vi "RPC_DAQ.vi"(7 "address":string[](array[string])=["192.168.10.20"], 8 "error in (no error)":errorcluster, 9 "stop":bool, 10 "save data":bool=TRUE, 11 "SMA mode":bool) -> (0 "error out 3":errorcluster, 2 "csv path":path=path "G:/tdc/2017/data/test_20250729_102001.csv", 3 "rate":dbl=0.9690537851551113)   [LabVIEW 2017]
uses:
  gloabal.vi
  <vilib>/Utility/file.llb/Write Delimited Spreadsheet (DBL).vi
  <vilib>/Utility/file.llb/Write Delimited Spreadsheet (I64).vi
panel:
  in  "index (row)":i32
  out "fine":u64
  out "Array 2":u64[](array[numeric])
  out "PAD":u64
  out "hitmap":u64=2 format="%08b"
  out "name (unnamed) 4":string
  out "name (unnamed) 3":string
  out "name (unnamed) 2":string
  out "Array":string[](array[string])
  out "pmt trigger rate":u32[](array[numeric])=[0, 59394, 0, 0, 0, 0, 0, 0, 0, 0, 0, 0, 0, 0, 0, 0, 0, 0, 0, 0, 0, 0, 0, 0, 0, 0, 0, 0, 0, 0, 0, 0, 0, 0, 0, 0, 0, 59424, 0, 0, 0, 0, 0, 0, 0, 0, 0, 0, 0, 0, 0, 0, 0, 0, 0, 0, 0, 0, 0, 0, 0, 0, 0, 0, 0, 0, 0, 0, 0, 0, 0, 0, 0, 0, 0, 0, 0, 0, 0, 0, 0, 0, 0, 0, 0, 0, 0, 0, 0, 0, 0, 0, 0, 0, 0, 0, 0, 0, 0, 0, 0, 0, 0, 0, 0, 0, 0, 0, 0, 0, 0, 0, 0, 0, 0, 0, 0, 0, 0, 0, 0, 0, 0, 0, 0, 0, 0, 0]
  out "event":u32[](array[numeric])=[0, 1657, 0, 0, 0, 0, 0, 0, 0, 0, 0, 0, 0, 0, 0, 0, 0, 0, 0, 0, 0, 0, 0, 0, 0, 0, 0, 0, 0, 0, 0, 0, 0, 0, 0, 0, 0, 863, 0, 0, 0, 0, 0, 0, 0, 0, 0, 0, 0, 0, 0, 0, 0, 0, 0, 0, 0, 0, 0, 0, 0, 0, 0, 0, 0, 0, 0, 0, 0, 0, 0, 0, 0, 0, 0, 0, 0, 0, 0, 0, 0, 0, 0, 0, 0, 0, 0, 0, 0, 0, 0, 0, 0, 0, 0, 0, 0, 0, 0, 0, 0, 0, 0, 0, 0, 0, 0, 0, 0, 0, 0, 0, 0, 0, 0, 0, 0, 0, 0, 0, 0, 0, 0, 0, 0, 0, 0, 0]
  in  "calib_file":path=path "G:/tdc/2017/data/112_20250410_codeDensity.csv" caption="文件路径 （空时为对话框）"
  in  "use_calib_file":bool
  in  "coarse counter width":u16(ring) items=["29", "48"]
  out "name (unnamed)":string
  out "error out 5":errorcluster
  in  "timeout":dbl=30000.0
  out "DAC":dbl=8094.0
  out "Out":u8=3 format="%.0x"
  in  "gps":bool
  out "Year":string="2025"
  in  "factor":i32=128
  in  "displayCR":bool=TRUE
  in  "Counter Setting":dbl=100000.0 format="%#_13g"
  in  "replace dat":bool
  in  "append csv":bool=TRUE
  out "element":string
  out "time":u64=1569737306459 format="%x"
  in  "UDP Config":bool
  in  "data  path":path=path "G:/tdc/2017/data"
  out "cal 2":u64[](graph)
  in  "Thresholds (mV)":dbl[](array[numeric])=[580.0, 580.0, 580.0, 580.0, 600.0, 600.0, 600.0, 600.0, 580.0, 580.0, 600.0, 600.0, 600.0, 600.0, 600.0, 600.0, 580.0, 580.0, 600.0, 600.0, 600.0, 600.0, 600.0, 600.0, 580.0, 580.0, 600.0, 600.0, 600.0, 600.0, 600.0, 600.0, 600.0, 600.0, 600.0, 600.0, 600.0, 600.0, 600.0, 600.0, 600.0, 600.0, 600.0, 600.0, 600.0, 600.0, 600.0, 600.0, 600.0, 600.0, 600.0, 600.0, 600.0, 600.0, 600.0, 600.0, 600.0, 600.0, 600.0, 600.0, 600.0, 600.0, 600.0, 600.0]
  out "error out 2":errorcluster
  in  "display":bool=TRUE
  in  "Thresholds":dbl=-0.03
  in  "one key for threshold":bool=TRUE
  in  "RST":bool
  in  "通道数量":i32=128
  out "Cal Table":u32[](array[numeric])
  in  "channel for cal":i32
  out "channel number":u64=1
  out "Calibration Counter":i32=3364
  out "Event index":i32=97959
  out "cal":i64[](graph)
  out "error out":errorcluster={"status"=TRUE, "code"=1, "source"="Close File in RPC_DAQ.vi"}
  out "appended path":path=path "G:/tdc/2017/data/test_20250729_102001.dat"
  in  "filename":string="test"
  in  "Events":i32=110000 min=1
  in  "timeout (ms)":i32=10000
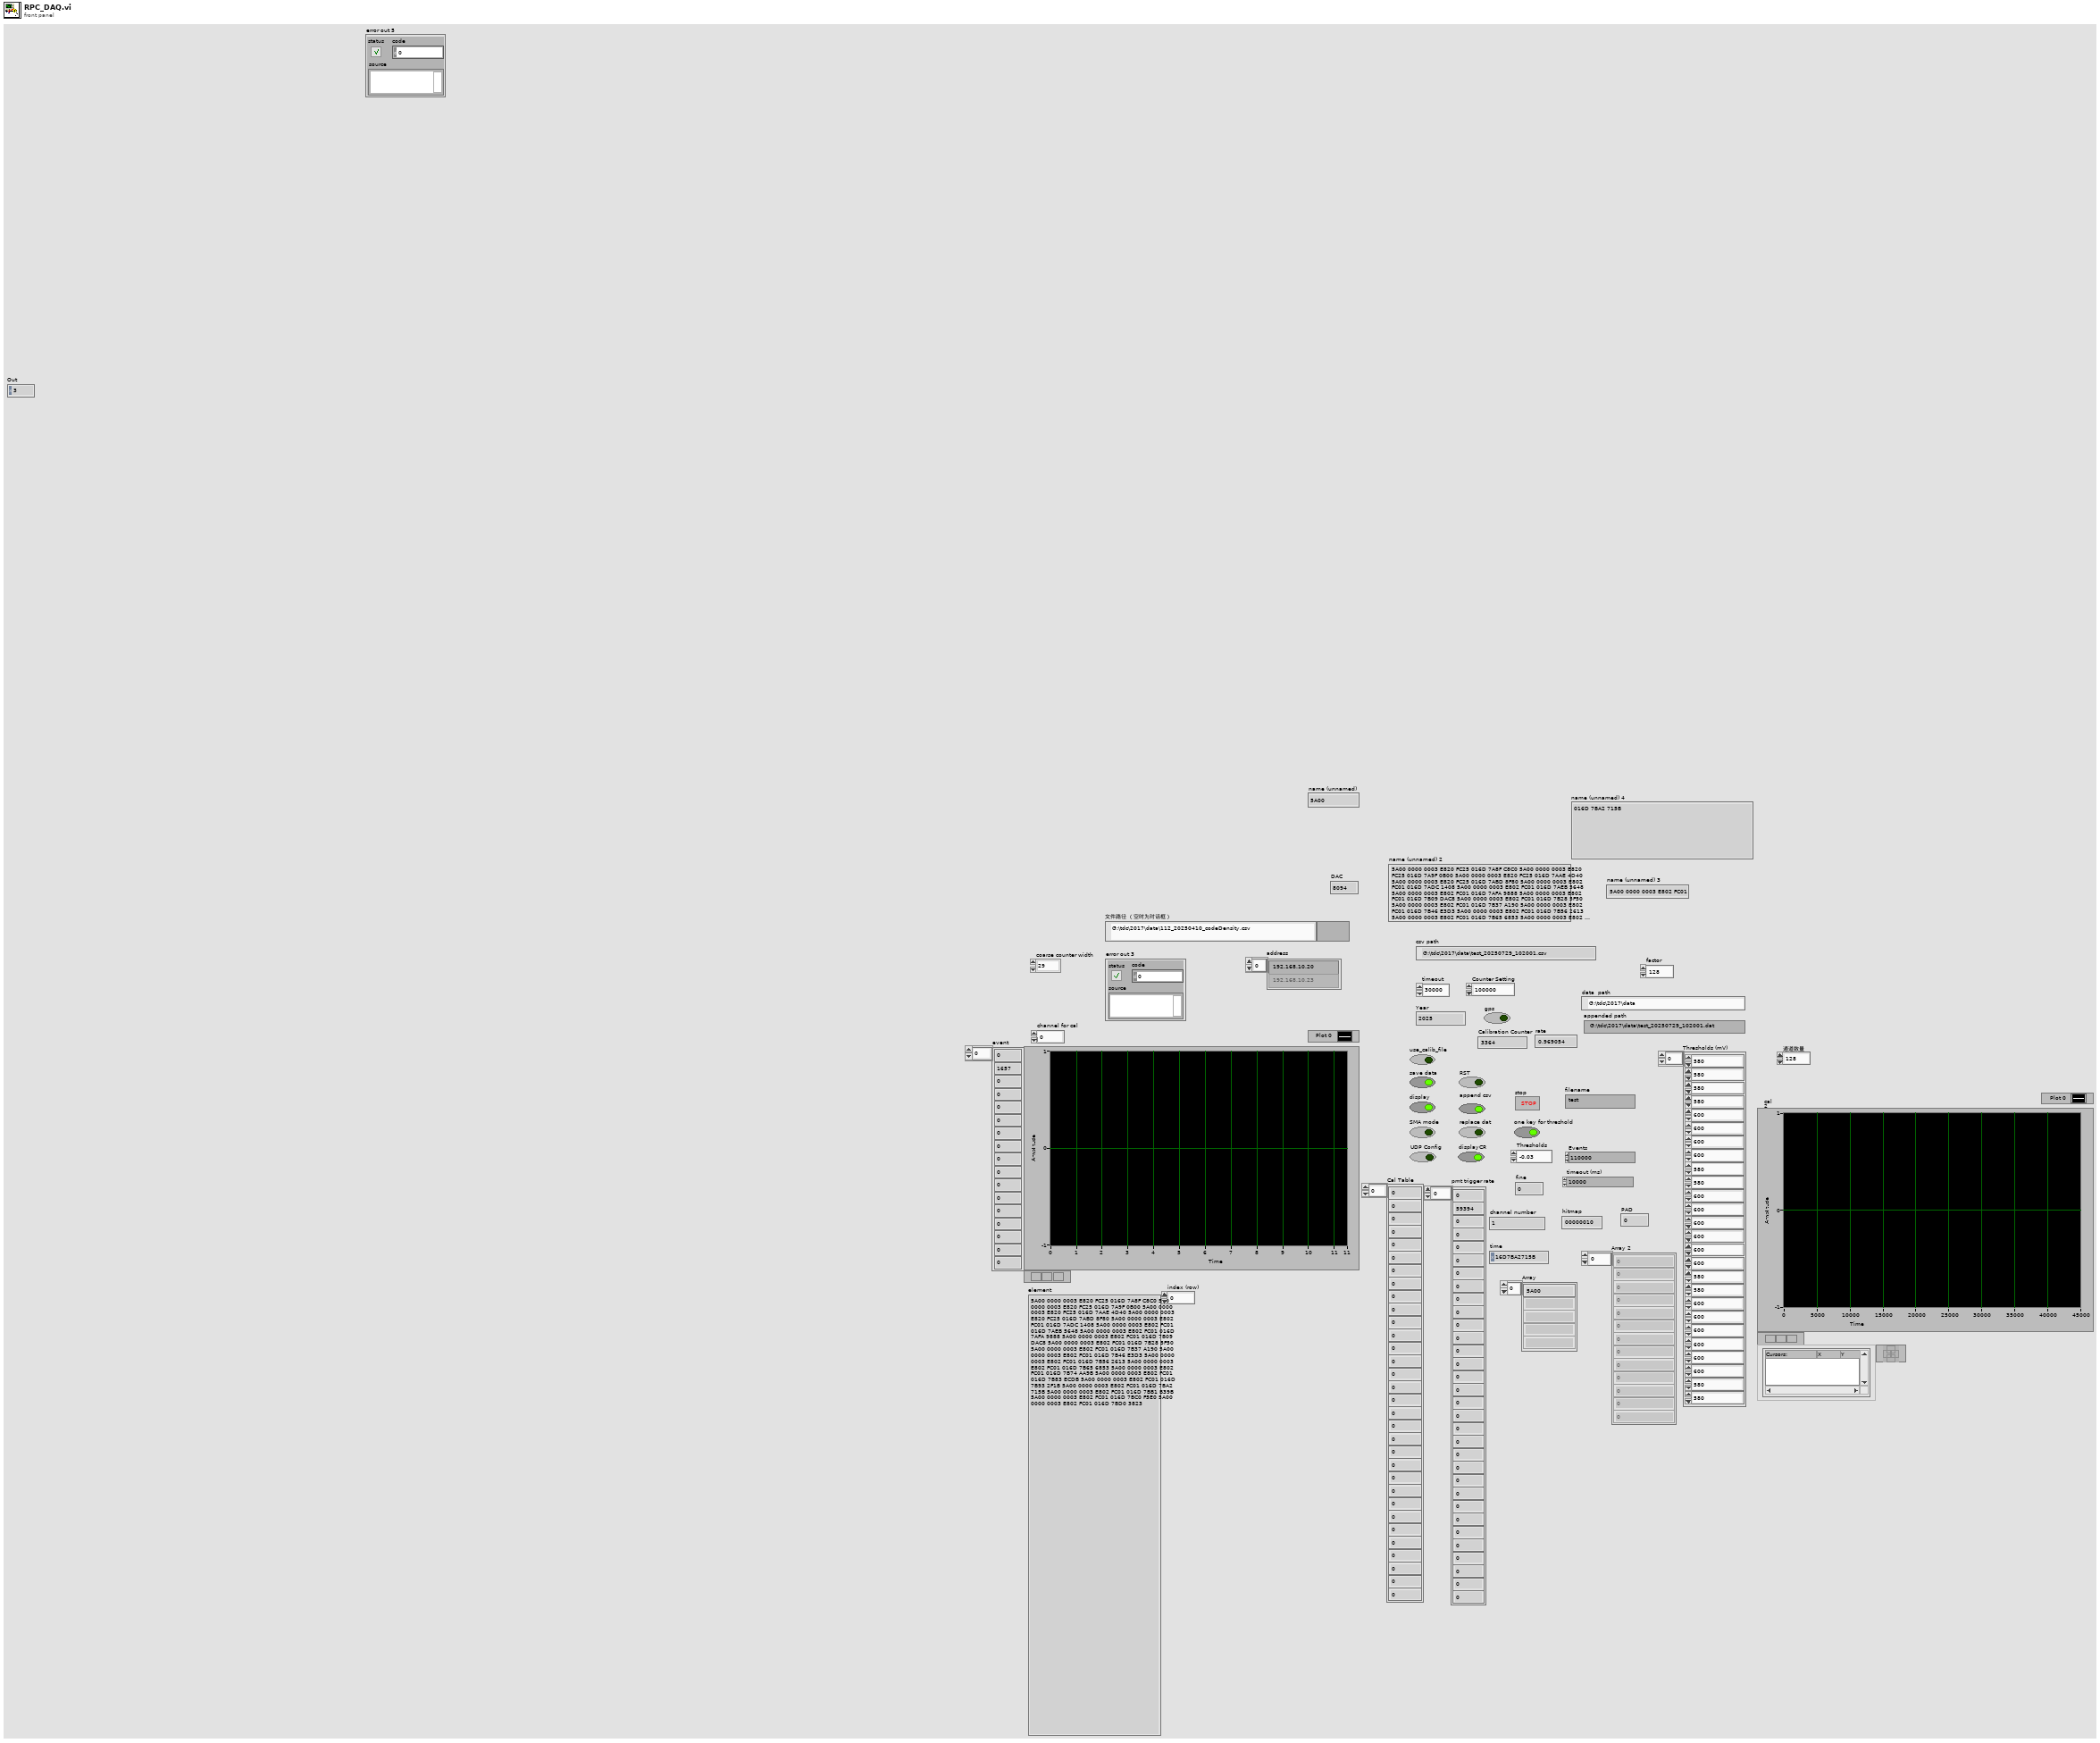
[diagram p1: front panel]
types:
  T1 = enum16{"open", "replace", "create", "open or create", "replace or create", "replace or create with confirmation"}
  T2 = enum16{"big-endian, network order", "native, host order", "little-endian"}
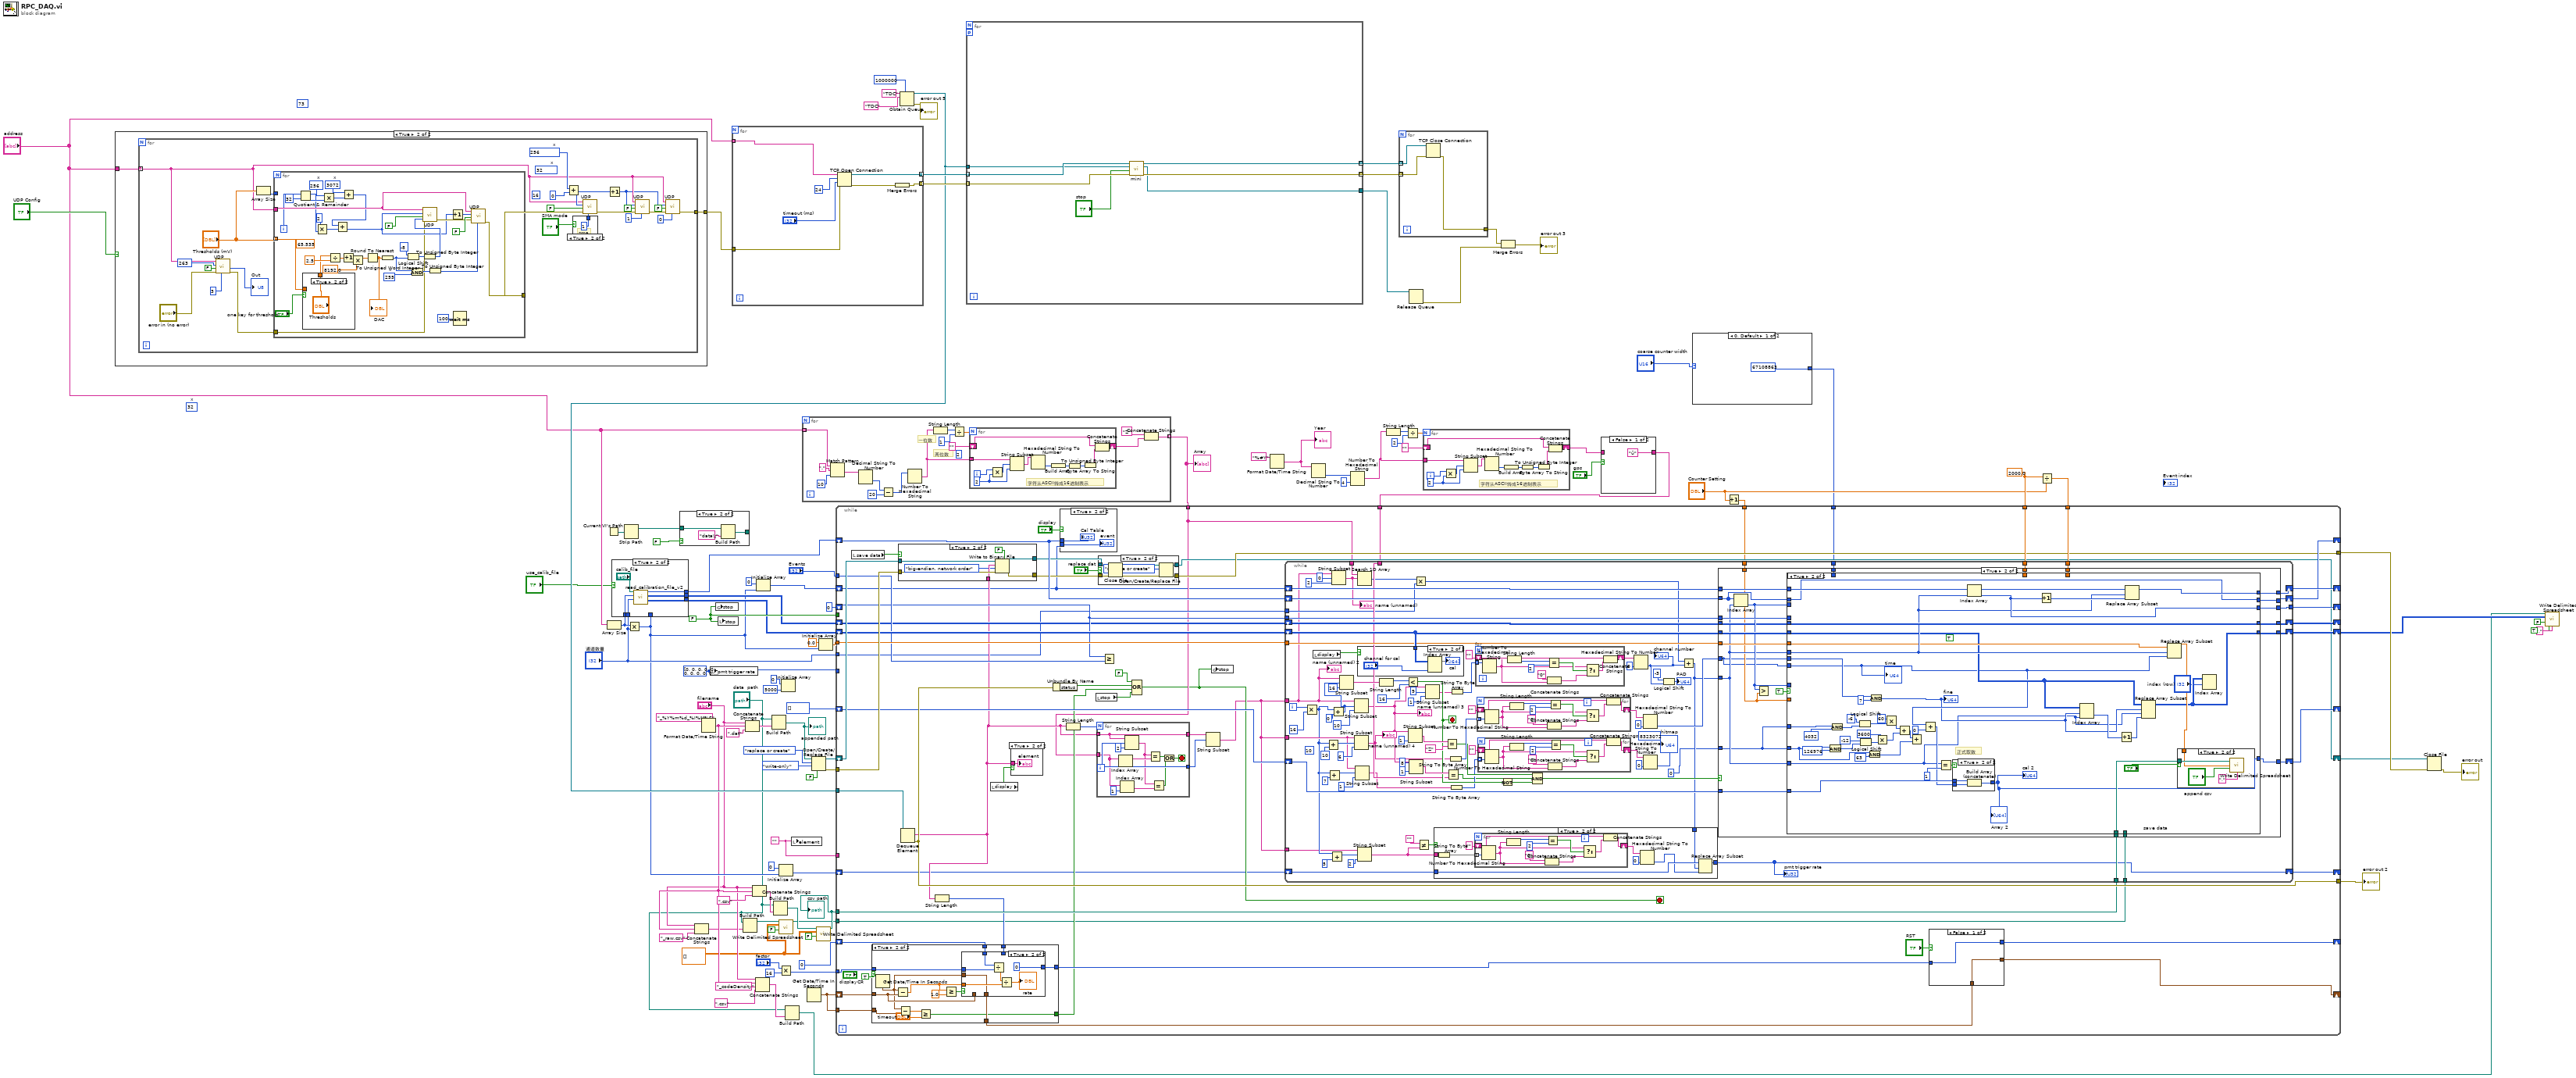
[diagram p0: block diagram]
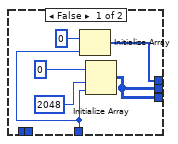
[diagram p2: hidden frame]
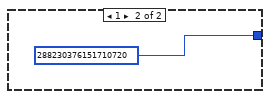
[diagram p3: hidden frame]
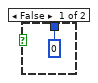
[diagram p6: hidden frame]
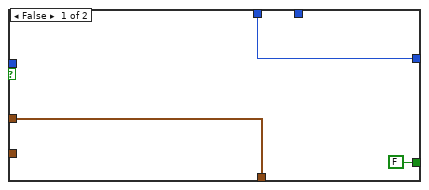
[diagram p12: hidden frame]
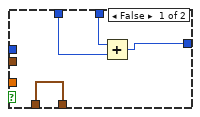
[diagram p13: hidden frame]
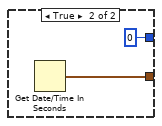
[diagram p15: hidden frame]
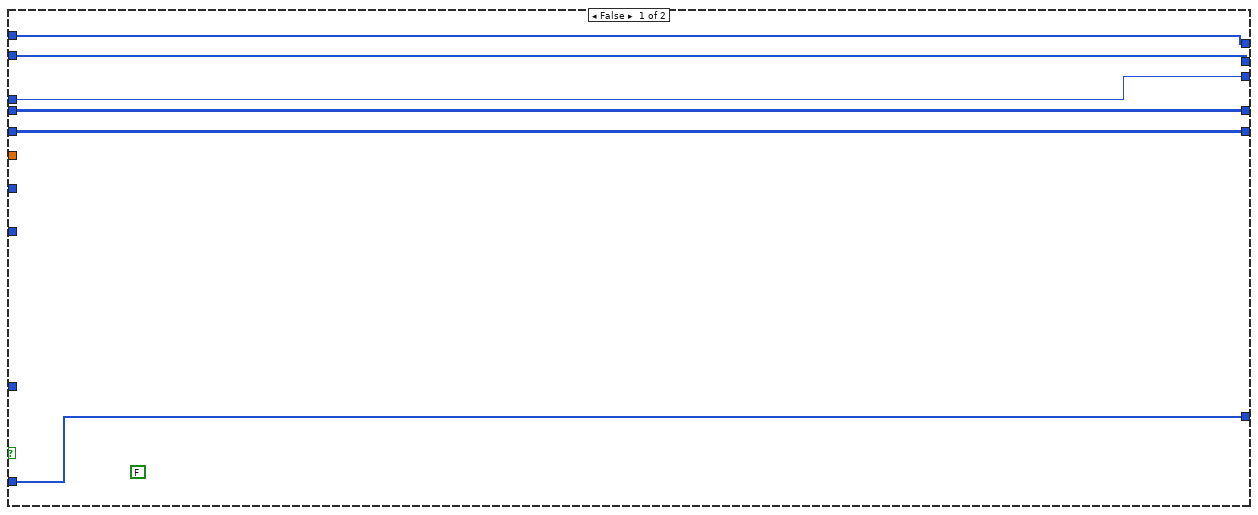
[diagram p18: hidden frame]
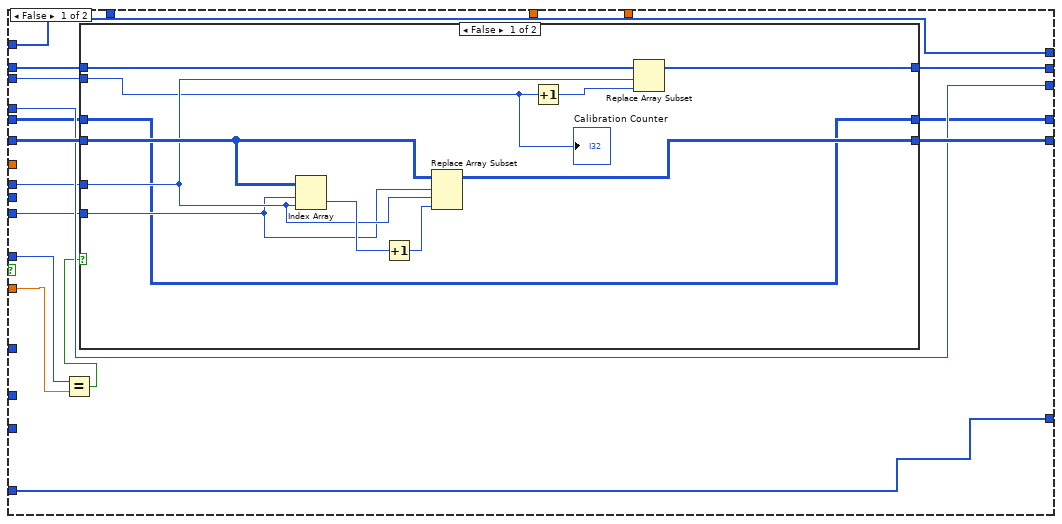
[diagram p19: hidden frame]
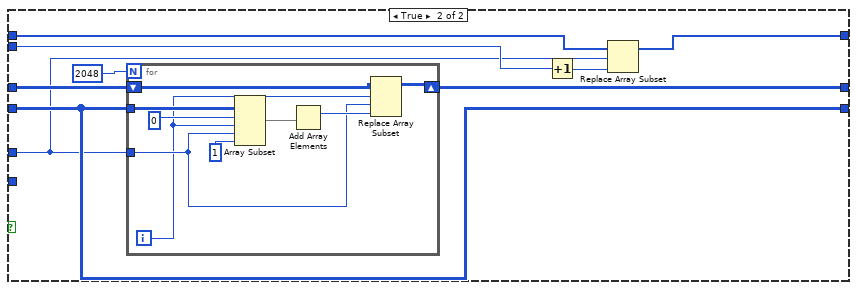
[diagram p20: hidden frame]
diagram:
  w11 = ""
  w12 = u32[] [0, 0, 0, 0, 0, 0, 0, 0, 0, 0, 0, 0, 0, 0, 0, 0, 0, 0, 0, 0, 0, 0, 0, 0, 0, 0, 0, 0, 0, 0, 0, 0, 0, 0, 0, 0, 0, 0, 0, 0, 0, 0, 0, 0, 0, 0, 0, 0, 0, 0, 0, 0, 0, 0, 0, 0, 0, 0, 0, 0, 0, 0, 0, 0] ("pmt trigger rate")
  (unwired) u32 73 ("Address")
  w63 = 2000.0 ("x")
  (unwired) u16 32  # x
  w25 = FALSE ("stop")
  w5 = dbl[][] [] ("2D data")
  n1 = case shown="True" "UDP Config" {
    tunnel: "address" -> [_ w100]
    tunnel: [_ w101] -> w30
    frame False {
    }
    frame True {
      n2 = for {
        tunnel: [w106] -> w101
        tunnel: w100 -> [w104] mode=indexing
        (unwired) u16 32  # x
        (unwired) u32 16 ("Address")
        w118 = u16 256  # x
        n3 = call "UDP.vi"("In"=u8 3, "error in (no error)"="error in (no error)", "Read (TRUE)"=FALSE, "Address"=u32 263, "IP address"=w104) -> ("error out"=w112:errorcluster, "Out"=→"Out":u8)  [unwired: 3 in, 1 out]
        n4 = Array Size(array="Thresholds (mV)") -> (size(s)=w121:i32)
        n5 = for {
          tunnel: w104 -> [w157]
          tunnel: "Thresholds (mV)" -> [w144] mode=indexing
          tunnel: [w147] -> w124
          tunnel: w121 -> [_]
          tunnel: w112 -> [w131]
          i -> [w139]
          (unwired) 65.535 ("y")
          w140 = u16 3072  # x
          w141 = u16 256  # x
          w153 = u16 255  # x
          n6 = Quotient & Remainder(x=w139, y=32) -> (x-y*floor(x/y)=w133:i32, floor(x/y)=w142:i32)
          n7 = case shown="True" "one key for threshold" {
            tunnel: [w163 "Thresholds"] -> w145
            tunnel: w144 -> [w163 _]
            frame False {
            }
            frame True {
            }
          }
          n8 = Multiply(x=2, y=w133) -> (x*y=w134:i32)
          n9 = Multiply(x=w141, y=w142) -> (x*y=w136:i32)
          n10 = Divide(x=w145, y=2.5) -> (x/y=w160:dbl)
          n11 = Increment(x=w160) -> (x+1=w130:dbl)
          n12 = Add(x=w140, y=w136) -> (x+y=w135:i32)
          n13 = Add(x=w135, y=w134) -> (x+y=w138:i32)
          n14 = Multiply(x=w130, y=8192.0) -> (x*y=w129:dbl)
          n15 = Round To Nearest(number=w129) -> (nearest integer value=w158:dbl)
          "DAC" <- w158
          n16 = To Unsigned Word Integer(number=w158) -> (unsigned 16bit integer=w149:u16)
          n17 = Logical Shift(y=i16 -8, x=w149) -> (x << y=w155:u16)
          n18 = And(x=w149, y=w153) -> (x .and. y?=w152:u16)
          n19 = To Unsigned Byte Integer(number=w155) -> (unsigned 8bit integer=w154:u8)
          n20 = call "UDP.vi"("In"=w154, "error in (no error)"=w131, "Read (TRUE)"=FALSE, "Address"=w138, "IP address"=w157) -> ("error out"=w148:errorcluster)  [unwired: 3 in, 2 out]
          n21 = To Unsigned Byte Integer(number=w152) -> (unsigned 8bit integer=w151:u8)
          n22 = Increment(x=w138) -> (x+1=w137:i32)
          n23 = Wait (ms)(milliseconds to wait=u32 100) -> ()  [unwired: 1 out]
          n24 = call "UDP.vi"("In"=w151, "error in (no error)"=w148, "Read (TRUE)"=FALSE, "Address"=w137, "IP address"=w157) -> ("error out"=w147:errorcluster)  [unwired: 3 in, 2 out]
        }
        n25 = Add(x=w118, y=u32 0 ("Address")) -> (x+y=w110:u32)
        n26 = case shown="True" "SMA mode" {
          tunnel: [u8 0 ("In") u8 1 ("In")] -> w123
          frame False {
          }
          frame True {
            # "sma"
          }
        }
        n27 = call "UDP.vi"("In"=w123, "error in (no error)"=w124, "Read (TRUE)"=FALSE, "Address"=w110, "IP address"=w104) -> ("error out"=w111:errorcluster)  [unwired: 3 in, 2 out]
        n28 = Increment(x=w110) -> (x+1=w103:u32)
        n29 = call "UDP.vi"("In"=u8 1, "error in (no error)"=w111, "Read (TRUE)"=FALSE, "Address"=w103, "IP address"=w104) -> ("error out"=w107:errorcluster)  [unwired: 3 in, 2 out]
        n30 = call "UDP.vi"("In"=u8 0, "error in (no error)"=w107, "Read (TRUE)"=FALSE, "Address"=w103, "IP address"=w104) -> ("error out"=w106:errorcluster)  [unwired: 3 in, 2 out]
      }
    }
  }
  n31 = Current VI's Path() -> (path=w94:path)
  n32 = Array Size(array="address") -> (size(s)=w17:i32)
  n33 = Strip Path(path=w94) -> (stripped path=w93:path)  [unwired: 1 out]
  n34 = Multiply(x=w17, y="通道数量") -> (x*y=w14:i32)
  n35 = case shown="True" "use_calib_file" {
    tunnel: w14 -> [w168 _]
    tunnel: [w165 w176] -> w20
    tunnel: [w165 w175] -> w19
    tunnel: [w166 w174] -> w18
    tunnel: w17 -> [_ w173]
    tunnel: "通道数量" -> [_ w172]
    frame False {
      n36 = Initialize Array(u32 0 ("element"), w168) -> (w166:u32[])
      n37 = Initialize Array(u32 0 ("element"), 2048 ("dimension size"), w168) -> (w165:u32[][])
    }
    frame True {
      n38 = call "read_calibration_file_v2.vi"("通道数量"=w172, "板子数量"=w173, "file path (dialog if empty)"="calib_file") -> ("code_density"=w176:i64[][], "accumulation"=w175:u32[][], "Cal Table"=w174:u32[])  [unwired: 5 in, 1 out]
    }
  }
  n39 = case shown="True" FALSE {
    tunnel: w93 -> [w177 w179]
    tunnel: [w177 w178] -> _
    frame False {
    }
    frame True {
      n40 = Build Path(base path=w179, name or relative path="data\\") -> (appended path=w178:path)
    }
  }
  n41 = Format Date/Time String(time format string (%c)="_%Y%m%d_%I%M%S") -> (date/time string=w9:string)  [unwired: 2 in]
  n42 = Concatenate Strings("filename", w9, "_raw.csv") -> (w7:string)
  n43 = local write "pmt trigger rate"(w12) -> ()
  n44 = global write "gloabal.vi" "stop"(w25) -> ()
  n45 = local write "stop"(w25) -> ()
  n46 = for {
    tunnel: "address" -> [w186] mode=indexing
    tunnel: [w185] -> w40 mode=indexing
    tunnel: [w183] -> w39 mode=indexing
    tunnel: w30 -> [w182]
    n47 = TCP Open Connection(address=w186, remote port or service name=u16 24 ("port"), timeout ms (60000)="timeout (ms)", error in (no error)=w182) -> (connection ID=w185:refnum<k5>, error out=w184:errorcluster)  [unwired: 1 in]
    n48 = Merge Errors(w184) -> (w183:errorcluster)
  }
  n49 = Build Path(base path="data  path", name or relative path=w7) -> (appended path=w2:path)
  n50 = Concatenate Strings("filename", w9, ".dat") -> (w92:string)
  n51 = Concatenate Strings("filename", w9, ".csv") -> (w82:string)
  n52 = Concatenate Strings("filename", w9, "_codeDensity" ("string"), ".csv") -> (w75:string)
  n53 = Initialize Array(u32 0 ("element"), w14) -> (w81:u32[])
  n54 = Build Path(base path="data  path", name or relative path=w92) -> (appended path=w91:path)
  "appended path" <- w91
  n55 = Build Path(base path="data  path", name or relative path=w82) -> (appended path=w80:path)
  n56 = Initialize Array(u32 0 ("element"), w14) -> (w13:u32[])
  n57 = call-poly <vilib>:"Write Delimited Spreadsheet.vi"("file path (dialog if empty)"=w2, "2D data"=w5, "append to file? (new file:F)"=FALSE) -> ("new file path (Not A Path if cancelled)"=w3:path)  [unwired: 11 in, 1 out]
  n58 = Multiply(x="factor", y=16) -> (x*y=w56:i32)
  n59 = Initialize Array(u32 0 ("element"), 5000 ("dimension size")) -> ()  [unwired: 1 out]
  n60 = Build Path(base path="data  path", name or relative path=w75) -> (appended path=w72:path)
  n61 = local write "element"(w11) -> ()
  n62 = for {
    tunnel: [w189] -> w42 mode=indexing
    tunnel: "address" -> [w188] mode=indexing
    (unwired) 2 ("y")
    # "一位数"
    # "两位数"
    n63 = Match Pattern(string=w188, regular expression="." ("search string"), offset (0)=10) -> (after substring=w195:string)  [unwired: 3 out]
    n64 = Decimal String To Number(string=w195) -> (number=w192:i32)  [unwired: 2 in, 1 out]
    n65 = Subtract(x=w192, y=20) -> (x-y=w191:i32)
    n66 = Number To Hexadecimal String(2:w191) -> (0:w194:string)  [unwired: 1 in]
    n67 = String Length(string=w194) -> (length=w200:i32)
    n68 = Divide(x=w200, y=1) -> (x/y=w201:dbl)
    n69 = for {
      N: w201 -> [_]
      shift-right: [w213] -> w190
      shift-left: "" ("format string") -> [w212]
      tunnel: w194 -> [w203]
      i -> [w211]
      w205 = 2 ("y")
      # "字符从ASCII转成16进制表示"
      n70 = Multiply(x=w211, y=w205) -> (x*y=w204:i32)
      n71 = String Subset(string=w203, offset (0)=w204, length (rest)=w205) -> (substring=w206:string)
      n72 = Hexadecimal String To Number(string=w206) -> (number=w210:u32)  [unwired: 2 in, 1 out]
      n73 = Build Array(w210) -> (w209:u32[])
      n74 = To Unsigned Byte Integer(number=w209) -> (unsigned 8bit integer=w208:u8[])
      n75 = Byte Array To String(unsigned byte array=w208) -> (string=w207:string)
      n76 = Concatenate Strings(w212, w207) -> (w213:string)
    }
    n77 = Concatenate Strings("Z", w190) -> (w189:string)
  }
  "Array" <- w42
  n78 = Get Date/Time In Seconds() -> (seconds since 1Jan1904=w41:timestamp)
  n79 = Open/Create/Replace File(file path (use dialog)=w91, operation (0:open)=T1."replace or create", access (0:read/write)=enum16{"read/write", "read-only", "write-only"}."write-only", disable buffering (F)=FALSE) -> (refnum out=w96:refnum<file>, error out=w95:errorcluster)  [unwired: 2 in, 1 out]
  n80 = call-poly <vilib>:"Write Delimited Spreadsheet.vi"("file path (dialog if empty)"=w80, "2D data"=w5, "append to file? (new file:F)"=FALSE) -> ("new file path (Not A Path if cancelled)"=w24:path)  [unwired: 11 in, 1 out]
  "csv path" <- w24
  n81 = Initialize Array(0.0, w14) -> (w68:dbl[])
  n82 = Obtain Queue(max queue size (-1, unlimited)=1000000, name (unnamed)="TDC", element data type="TDC" ("name (unnamed)")) -> (queue out=w31:refnum<queue>, error out=→"error out 5":errorcluster)  [unwired: 2 in, 1 out]
  n83 = for {
    tunnel: w40 -> [w220] mode=indexing
    tunnel: w39 -> [w219] mode=indexing
    tunnel: [w218] -> w38 mode=indexing
    tunnel: [w217] -> w37 mode=indexing
    workers-P: _ -> [_]
    tunnel: w31 -> [w216]
    tunnel: [w215] -> w32
    n84 = call "mini.vi"("error in (no error)"=w219, "stop"="stop", "queue out 2"=w216, "connection ID 2"=w220) -> ("error out 3"=w217:errorcluster, "queue out"=w215:refnum<queue>, "connection ID"=w218:refnum<k5>)  [unwired: 5 in]
  }
  n85 = Format Date/Time String(time format string (%c)="%#Y") -> (date/time string=w53:string)  [unwired: 2 in]
  "Year" <- w53
  n86 = Decimal String To Number(string=w53) -> (number=w52:i32)  [unwired: 2 in, 1 out]
  n87 = Number To Hexadecimal String(1:i16 4 ("width (-)"), 2:w52) -> (0:w46:string)
  n88 = String Length(string=w46) -> (length=w48:i32)
  n89 = for {
    tunnel: w38 -> [w223] mode=indexing
    tunnel: w37 -> [w222] mode=indexing
    tunnel: [w221] -> w29
    n90 = TCP Close Connection(connection ID=w223, error in (no error)=w222) -> (error out=w221:errorcluster)  [unwired: 1 in, 1 out]
  }
  n91 = Divide(x=w48, y=2) -> (x/y=w49:dbl)
  n92 = Release Queue(queue=w32) -> (error out=w28:errorcluster)  [unwired: 2 in, 2 out]
  n93 = for {
    N: w49 -> [_]
    shift-right: [w234] -> w45
    shift-left: "" ("format string") -> [w233]
    tunnel: w46 -> [w224]
    i -> [w232]
    w226 = 2 ("y")
    # "字符从ASCII转成16进制表示"
    n94 = Multiply(x=w232, y=w226) -> (x*y=w225:i32)
    n95 = String Subset(string=w224, offset (0)=w225, length (rest)=w226) -> (substring=w227:string)
    n96 = Hexadecimal String To Number(string=w227) -> (number=w231:u32)  [unwired: 2 in, 1 out]
    n97 = Build Array(w231) -> (w230:u32[])
    n98 = To Unsigned Byte Integer(number=w230) -> (unsigned 8bit integer=w229:u8[])
    n99 = Byte Array To String(unsigned byte array=w229) -> (string=w228:string)
    n100 = Concatenate Strings(w233, w228) -> (w234:string)
  }
  n101 = Merge Errors(w29, w28) -> (→"error out 3":errorcluster)
  n102 = case shown="False" "gps" {
    tunnel: w45 -> [_ w236]
    tunnel: ["ü" ("format string") w236] -> w44
    frame False {
    }
    frame True {
    }
  }
  n103 = case shown="0, Default" "coarse counter width" {
    tunnel: [u64 67108863 ("port") u64 288230376151710720 ("port")] -> w22
    frame 0, Default {
    }
    frame 1 {
    }
  }
  n104 = Increment(x="Counter Setting") -> (x+1=w59:dbl)
  n105 = Divide(x=w63, y="Counter Setting") -> (x/y=w62:dbl)
  n106 = while {
    tunnel: w95 -> [w296]
    tunnel: [w277] -> w69
    tunnel: [w266] -> w88
    shift-right: [w293] -> w73
    shift-left: w20 -> [w294]
    tunnel: "Events" -> [w291]
    shift-right: [w290] -> _
    shift-left: w81 -> [w243]
    shift-right: [w289] -> _
    shift-left: u32 0 ("element") -> [w288]
    shift-right: [w287] -> _
    shift-left: w18 -> [w279]
    shift-right: [w281] -> _
    shift-left: w19 -> [w286]
    tunnel: w24 -> [w273]
    shift-right: [w285] -> _
    shift-left: 0 -> [w260]
    shift-right: [w283] -> _
    shift-left: w41 -> [w282]
    tunnel: w25 -> [_]
    tunnel: w31 -> [w278]
    shift-right: [w274] -> _
    shift-left: u64[] [] -> [w275]
    tunnel: w42 -> [w247]
    tunnel: w63 -> [w271]
    tunnel: w62 -> [w270]
    shift-right: [w265] -> w61
    shift-left: w96 -> [w295]
    tunnel: w59 -> [w264]
    tunnel: w56 -> [w257]
    tunnel: w44 -> [w255]
    tunnel: w41 -> [w254]
    tunnel: "通道数量" -> [w248]
    tunnel: w22 -> [w244]
    shift-right: [w240] -> _
    shift-left: w13 -> [w241]
    tunnel: w12 -> [_]
    tunnel: w11 -> [_]
    tunnel: w3 -> [w239]
    tunnel: w68 -> [w292]
    stop <- w246 stop-if-true
    n107 = local read "save data"() -> (w259:bool)
    n108 = Dequeue Element(queue=w278) -> (element=w250:string, error out=w277:errorcluster)  [unwired: 2 in, 2 out]
    n109 = case shown="True" w259 {
      tunnel: w296 -> [w309 w317]
      tunnel: w295 -> [w310 w316]
      tunnel: w250 -> [_ w314]
      tunnel: [w310 w313] -> w269
      tunnel: [w309 w312] -> w267
      frame False {
      }
      frame True {
        n110 = Write to Binary File(file (use dialog)=w316, data=w314, error in=w317, 5:FALSE ("prepend array or string size? (T)"), 9:T2."big-endian, network order" ("byte order (0:big-endian, network order)")) -> (refnum out=w313:refnum<file>, error out=w312:errorcluster)  [unwired: 1 in, 1 out]
      }
    }
    n111 = String Length(string=w250) -> (length=w261:i32)
    n112 = case shown="True" TRUE {
      tunnel: w282 -> [w329 w339]
      tunnel: [w329 w340] -> w263
      tunnel: w260 -> [w328 w338]
      tunnel: w261 -> [_ w337]
      tunnel: [w328 w336] -> w262
      tunnel: w257 -> [_ w335]
      tunnel: w254 -> [_ w333]
      tunnel: [FALSE w330] -> w253
      frame False {
      }
      frame True {
        n113 = Get Date/Time In Seconds() -> (seconds since 1Jan1904=w334:timestamp)
        n114 = Subtract(x=w334, y=w339) -> (x-y=w342:dbl)
        n115 = Subtract(x=w334, y=w333) -> (x-y=w332:dbl)
        n116 = Greater Or Equal?(x=w332, y="timeout") -> (x >= y?=w330:bool)
        n117 = Greater Or Equal?(x=w342, y=1.0) -> (x >= y?=w343:bool)
        n118 = case shown="True" w343 {
          tunnel: w342 -> [_ w354]
          tunnel: w334 -> [_ w352]
          tunnel: [w347 w352] -> w340
          tunnel: w339 -> [w347 _]
          tunnel: w338 -> [w346 w349]
          tunnel: w337 -> [w345 _]
          tunnel: [w344 0] -> w336
          tunnel: w335 -> [_ w348]
          frame False {
            n119 = Add(x=w345, y=w346) -> (x+y=w344:i32)
          }
          frame True {
            n120 = Divide(x=w349, y=w348) -> (x/y=w351:dbl)
            n121 = Divide(x=w351, y=w354) -> (x/y=→"rate":dbl)
          }
        }
      }
    }
    n122 = local read "display"() -> (w258:bool)
    n123 = case shown="True" w258 {
      tunnel: w250 -> [_ w308]
      frame False {
      }
      frame True {
        "element" <- w308
      }
    }
    n124 = Unbundle By Name(w277) -> ("status"=w276:bool)
    n125 = case shown="True" "display" {
      tunnel: w279 -> [_ w356]
      tunnel: w243 -> [_ w355]
      frame False {
      }
      frame True {
        "Cal Table" <- w356
        "event" <- w355
      }
    }
    n126 = String Length(string=w250) -> (length=w252:i32)
    n127 = local read "stop"() -> (w245:bool)
    n128 = for {
      N: w252 -> [_]
      tunnel: w250 -> [w305]
      tunnel: [w305] -> w251
      tunnel: [w304] -> w249
      tunnel: w247 -> [w302]
      i -> [w304]
      stop <- w298 stop-if-true
      n129 = Index Array(array=w302) -> (element=w303:string)  [unwired: 1 in]
      n130 = Index Array(array=w302, index=1) -> (element=w300:string)
      n131 = String Subset(string=w305, offset (0)=w304, length (rest)=2 ("length (rest)")) -> (substring=w299:string)
      n132 = Equal?(x=w299, y=w303) -> (x = y?=w306:bool)
      n133 = Equal?(x=w299, y=w300) -> (x = y?=w297:bool)
      n134 = Or(x=w306, y=w297) -> (x .or. y?=w298:bool)
    }
    n135 = case shown="True" "replace dat" {
      tunnel: w269 -> [w319 w325]
      tunnel: [w319 w324] -> w265
      tunnel: w267 -> [w318 w321]
      tunnel: [w318 w320] -> w266
      frame False {
      }
      frame True {
        n136 = Close File(refnum=w325, error in=w321) -> (path=w326:path, error out=w322:errorcluster)
        n137 = Open/Create/Replace File(file path (use dialog)=w326, error in=w322, operation (0:open)=T1."replace or create") -> (refnum out=w324:refnum<file>, error out=w320:errorcluster)  [unwired: 3 in, 1 out]
      }
    }
    n138 = Greater Or Equal?(x=w288, y=w291) -> ()  [unwired: 1 out]
    n139 = Compound Arithmetic op=OR(FALSE ("x"), w276, w253, w245) -> (w246:bool)
    n140 = String Subset(string=w251, offset (0)=w249) -> (substring=w242:string)  [unwired: 1 in]
    n141 = global write "gloabal.vi" "stop"(w246) -> ()
    n142 = while {
      tunnel: w242 -> [w369]
      shift-right: [w448] -> w293
      shift-left: w294 -> [w447]
      shift-right: [w443] -> w290
      shift-left: w243 -> [w442]
      tunnel: [w441] -> w289
      tunnel: w288 -> [w440]
      shift-right: [w438] -> w287
      shift-left: w279 -> [w439]
      tunnel: w273 -> [w436]
      shift-right: [w435] -> w281
      shift-left: w286 -> [w406]
      shift-right: [w432] -> w274
      shift-left: w275 -> [w433]
      tunnel: w242 -> [w400]
      tunnel: w271 -> [w413]
      tunnel: w270 -> [w412]
      tunnel: w264 -> [w405]
      tunnel: w255 -> [w395]
      tunnel: w248 -> [w385]
      tunnel: w247 -> [w384]
      tunnel: w244 -> [w382]
      tunnel: w242 -> [w375]
      shift-right: [w366] -> w240
      shift-left: w241 -> [w377]
      tunnel: w239 -> [w371]
      tunnel: w292 -> [w446]
      i -> [w449]
      stop <- w408 stop-if-true
      (unwired) 10 ("length (rest)")
      (unwired) u64 8323072 ("port")
      n143 = Multiply(x=w449, y=16 ("length (rest)")) -> (x*y=w378:i32)
      n144 = local read "display"() -> (w434:bool)
      n145 = Add(x=w378, y=10 ("length (rest)")) -> (x+y=w424:i32)
      n146 = Add(x=w378, y=7 ("length (rest)")) -> (x+y=w402:i32)
      n147 = Add(x=w378, y=5 ("length (rest)")) -> (x+y=w380:i32)
      n148 = Add(x=w378, y=0 ("length (rest)")) -> (x+y=w411:i32)
      n149 = String Subset(string=w369, offset (0)=0, length (rest)=2 ("length (rest)")) -> (substring=w386:string)
      "name (unnamed)" <- w386
      n150 = String Subset(string=w369, offset (0)=w411, length (rest)=16 ("y")) -> (substring=w409:string)
      n151 = String Subset(string=w369, offset (0)=w411, length (rest)=10 ("length (rest)")) -> (substring=w368:string)
      "name (unnamed) 3" <- w368
      n152 = String Subset(string=w400, offset (0)=w424, length (rest)=6 ("length (rest)")) -> (substring=w367:string)
      "name (unnamed) 4" <- w367
      n153 = String Subset(string=w400, offset (0)=w402, length (rest)=1 ("length (rest)")) -> (substring=w391:string)
      n154 = Search 1D Array(1D array=w384, element=w386) -> (index of element=w387:i32)  [unwired: 1 in]
      n155 = case shown="True" w434 {
        tunnel: w447 -> [_ w494]
        frame False {
        }
        frame True {
          n156 = Index Array(array=w494, index (col)="channel for cal") -> (element=→"cal":i64[])  [unwired: 1 in]
        }
      }
      n157 = String Subset(string=w375, offset (0)=w380, length (rest)=2 ("length (rest)")) -> (substring=w373:string)
      n158 = String Length(string=w409) -> (length=w445:i32)
      n159 = Less?(x=w445, y=16) -> (x < y?=w408:bool)
      n160 = String Subset(string=w368, length (rest)=1 ("length (rest)")) -> (substring=w429:string)  [unwired: 1 in]
      n161 = String Subset(string=w368, offset (0)=8, length (rest)=1 ("length (rest)")) -> (substring=w414:string)
      n162 = Multiply(x=w387, y=w385) -> (x*y=w383:i32)
      n163 = Not Equal?(x="", y=w373) -> (x != y?=w374:bool)
      n164 = String Subset(string=w368, offset (0)=9, length (rest)=1 ("length (rest)")) -> (substring=w392:string)
      n165 = Equal?(x=w429, y="Z" ("format string")) -> (x = y?=w415:bool)
      n166 = Equal?(x=w414, y=w395) -> (x = y?=w365:bool)
      n167 = String To Byte Array(string=w367) -> (unsigned byte array=w421:u8[])
      n168 = String To Byte Array(string=w391) -> (unsigned byte array=w396:u8[])
      n169 = String To Byte Array(string=w392) -> (unsigned byte array=w450:u8[])
      n170 = for {
        shift-right: [w629] -> w418
        shift-left: "" ("format string") -> [w626]
        tunnel: w450 -> [w630] mode=indexing
        n171 = Number To Hexadecimal String(2:w630) -> (0:w622:string)  [unwired: 1 in]
        n172 = String Length(string=w622) -> (length=w628:i32)
        n173 = Equal?(x=w628, y=2) -> (x = y?=w625:bool)
        n174 = Concatenate Strings("0" ("format string"), w622) -> (w624:string)
        n175 = Select(t=w622, s=w625, f=w624) -> (s? t:f=w621:string)
        n176 = Concatenate Strings(w626, w621) -> (w629:string)
      }
      n177 = for {
        shift-right: [w490] -> w419
        shift-left: "" ("format string") -> [w482]
        tunnel: w421 -> [w491] mode=indexing
        n178 = Number To Hexadecimal String(2:w491) -> (0:w484:string)  [unwired: 1 in]
        n179 = String Length(string=w484) -> (length=w489:i32)
        n180 = Concatenate Strings("0" ("format string"), w484) -> (w486:string)
        n181 = Equal?(x=w489, y=2) -> (x = y?=w487:bool)
        n182 = Select(t=w484, s=w487, f=w486) -> (s? t:f=w483:string)
        n183 = Concatenate Strings(w482, w483) -> (w490:string)
      }
      n184 = for {
        shift-right: [w480] -> w399
        shift-left: "" ("format string") -> [w472]
        tunnel: w396 -> [w481] mode=indexing
        n185 = Number To Hexadecimal String(2:w481) -> (0:w474:string)  [unwired: 1 in]
        n186 = String Length(string=w474) -> (length=w479:i32)
        n187 = Concatenate Strings("0" ("format string"), w474) -> (w476:string)
        n188 = Equal?(x=w479, y=2) -> (x = y?=w477:bool)
        n189 = Select(t=w474, s=w477, f=w476) -> (s? t:f=w473:string)
        n190 = Concatenate Strings(w472, w473) -> (w480:string)
      }
      n191 = Not(x=w408) -> (.not. x?=w407:bool)
      n192 = Compound Arithmetic op=AND(w415, w365, w407) -> (w427:bool)
      n193 = Hexadecimal String To Number(string=w418, default (0uL)=u64 0 ("default (0 U32)")) -> (number=w362:u64)  [unwired: 1 in, 1 out]
      "channel number" <- w362
      n194 = Hexadecimal String To Number(string=w419, default (0uL)=u64 0 ("default (0 U32)")) -> (number=w390:u64)  [unwired: 1 in, 1 out]
      n195 = Hexadecimal String To Number(string=w399, default (0uL)=u64 0 ("default (0 U32)")) -> (number=→"hitmap":u64)  [unwired: 1 in, 1 out]
      n196 = Logical Shift(y=i16 -3, x=w362) -> (x << y=→"PAD":u64)
      n197 = Add(x=w383, y=w362) -> (x+y=w376:u64)
      n198 = case shown="True" w374 {
        tunnel: w377 -> [w452 w458]
        tunnel: w376 -> [_ w456]
        tunnel: [w452 w455] -> w366
        tunnel: w373 -> [_ w454]
        frame False {
        }
        frame True {
          n199 = String To Byte Array(string=w454) -> (unsigned byte array=w459:u8[])
          n200 = for {
            shift-right: [w470] -> w453
            shift-left: "" ("format string") -> [w462]
            tunnel: w459 -> [w471] mode=indexing
            n201 = Number To Hexadecimal String(2:w471) -> (0:w464:string)  [unwired: 1 in]
            n202 = String Length(string=w464) -> (length=w469:i32)
            n203 = Concatenate Strings("0" ("format string"), w464) -> (w466:string)
            n204 = Equal?(x=w469, y=2) -> (x = y?=w467:bool)
            n205 = Select(t=w464, s=w467, f=w466) -> (s? t:f=w463:string)
            n206 = Concatenate Strings(w462, w463) -> (w470:string)
          }
          n207 = Hexadecimal String To Number(string=w453, default (0uL)=u64 0 ("default (0 U32)")) -> (number=w457:u64)  [unwired: 1 in, 1 out]
          n208 = Replace Array Subset(array=w458, new element=w457, index=w456) -> (w455:u32[])
        }
      }
      "pmt trigger rate" <- w366
      n209 = case shown="True" w427 {
        tunnel: w390 -> [_ w501]
        tunnel: w440 -> [w498 w518]
        tunnel: w447 -> [w500 w524]
        tunnel: [w500 w523] -> w448
        tunnel: w446 -> [_ w522]
        tunnel: w376 -> [_ w509]
        tunnel: w442 -> [w499 w521]
        tunnel: [w499 w520] -> w443
        tunnel: [w498 w519] -> w441
        tunnel: w439 -> [w497 w517]
        tunnel: [w497 w516] -> w438
        tunnel: w406 -> [w496 w514]
        tunnel: [w496 w513] -> w435
        tunnel: w436 -> [_ w512]
        tunnel: w433 -> [w495 w511]
        tunnel: [w495 w510] -> w432
        tunnel: w413 -> [_ w508]
        tunnel: w412 -> [_ w507]
        tunnel: w405 -> [_ w506]
        tunnel: u64 0 ("default (0 U32)") -> [_ w505]
        tunnel: w382 -> [_ w504]
        tunnel: w371 -> [_ w503]
        frame False {
          (unwired) FALSE
        }
        frame True {
          n210 = Index Array(array=w517, index=w509) -> (element=w515:u32)
          n211 = Greater?(x=w515, y=w506) -> ()  [unwired: 1 out]
          n212 = case shown="True" TRUE {
            tunnel: w524 -> [w539 w574]
            tunnel: [w538 w572] -> w523
            tunnel: w501 -> [w531 w573]
            tunnel: w522 -> [_ w580]
            tunnel: w518 -> [w536 _]
            tunnel: w509 -> [w534 w581]
            tunnel: w521 -> [w537 w612]
            tunnel: [w537 w611] -> w520
            tunnel: [w536 w609] -> w519
            tunnel: w515 -> [w532 _]
            tunnel: w517 -> [w535 w608]
            tunnel: [w533 w608] -> w516
            tunnel: w515 -> [w529 _]
            tunnel: w506 -> [w526 _]
            tunnel: w514 -> [w528 w607]
            tunnel: [w527 w607] -> w513
            tunnel: w512 -> [_ w606]
            tunnel: w511 -> [w525 w603]
            tunnel: [w525 w602] -> w510
            tunnel: w509 -> [_ w569]
            tunnel: w508 -> [_ _]
            tunnel: w507 -> [_ _]
            tunnel: w505 -> [_ w596]
            tunnel: w505 -> [_ w585]
            tunnel: w501 -> [_ w579]
            tunnel: w504 -> [_ _]
            tunnel: w503 -> [_ _]
            frame False {
              n213 = Equal?(x=w529, y=w526) -> (x = y?=w530:bool)
              n214 = case shown="False" w530 {
                tunnel: w539 -> [w550 w556]
                tunnel: [w548 w556] -> w538
                tunnel: w535 -> [w546 w554]
                tunnel: w534 -> [w545 w551]
                tunnel: [w543 w553] -> w533
                tunnel: w532 -> [w542 w552]
                tunnel: w531 -> [w541 _]
                tunnel: w528 -> [w540 w558]
                tunnel: [w540 w557] -> w527
                frame False {
                  n215 = Index Array(array=w550, index (row)=w541, index (col)=w545) -> (element=w549:i64)
                  n216 = Increment(x=w549) -> (x+1=w547:i64)
                  n217 = Replace Array Subset(array=w550, new element=w547, index (row)=w541, index (col)=w545) -> (w548:i64[][])
                  n218 = Increment(x=w542) -> (x+1=w544:u32)
                  n219 = Replace Array Subset(array=w546, new element=w544, index=w545) -> (w543:u32[])
                  "Calibration Counter" <- w542
                }
                frame True {
                  n220 = for {
                    N: 2048 -> [_]
                    tunnel: w556 -> [w568]
                    tunnel: w551 -> [w561]
                    shift-right: [w563] -> w557
                    shift-left: w558 -> [w564]
                    i -> [w560]
                    n221 = Array Subset(array=w568, index (row)=0 ("索引"), length (row)=w560, index (col)=w561, length (col)=1 ("长度")) -> (w565:i64[][])
                    n222 = Add Array Elements(numeric array=w565) -> (sum=w562:i64)
                    n223 = Replace Array Subset(array=w564, new element=w562, index (row)=w560, index (col)=w561) -> (w563:u32[][])
                  }
                  n224 = Increment(x=w552) -> (x+1=w555:u32)
                  n225 = Replace Array Subset(array=w554, new element=w555, index=w551) -> (w553:u32[])
                }
              }
            }
            frame True {
              (unwired) TRUE
              # "正式取数"
              n226 = And(x=w585, y=u64 126976 ("port")) -> (x .and. y?=w593:u64)
              n227 = And(x=w596, y=u64 4032 ("port")) -> (x .and. y?=w599:u64)
              n228 = Logical Shift(y=i16 -6, x=w599) -> (x << y=w584:u64)
              n229 = Logical Shift(y=i16 -12, x=w593) -> (x << y=w592:u64)
              n230 = And(x=w585, y=u64 63 ("port")) -> (x .and. y?=w582:u64)
              n231 = And(x=w579, y=u64 7) -> (x .and. y?=w570:u64)
              "fine" <- w570
              n232 = Multiply(x=u64 3600, y=w592) -> (x*y=w588:u64)
              n233 = Multiply(x=u64 60, y=w584) -> (x*y=w589:u64)
              n234 = Add(x=w589, y=w588) -> (x+y=w587:u64)
              n235 = Add(x=w587, y=w582) -> ()  [unwired: 1 out]
              n236 = Add(x=w573, y=u64 0) -> (x+y=w583:u64)
              n237 = Equal?(x=w569, y=u32 1) -> (x = y?=w601:bool)
              n238 = case shown="True" w601 {
                tunnel: w603 -> [w613 w616]
                tunnel: w583 -> [_ w615]
                tunnel: [w613 w614] -> w602
                frame False {
                }
                frame True {
                  n239 = Build Array (concatenate)(w616, w615) -> (w614:u64[])
                }
              }
              "cal 2" <- w602
              "Array 2" <- w602
              n240 = Index Array(array=w612, index=w581) -> (element=w609:u32)
              n241 = Increment(x=w609) -> (x+1=w610:u32)
              n242 = Index Array(array=w574, index (row)=w570, index (col)=w569) -> (element=w576:i64)
              n243 = Increment(x=w576) -> (x+1=w575:i64)
              n244 = Replace Array Subset(array=w612, new element=w610, index=w581) -> (w611:u32[])
              n245 = Replace Array Subset(array=w574, new element=w575, index (row)=w570, index (col)=w569) -> (w572:i64[][])
              n246 = Replace Array Subset(array=w580, new element=w573, index=w581) -> (w605:dbl[])
              n247 = case shown="True" "save data" {
                tunnel: w606 -> [_ w620]
                tunnel: w605 -> [_ w618]
                frame False {
                }
                frame True {
                  n248 = call-poly <vilib>:"Write Delimited Spreadsheet.vi"("file path (dialog if empty)"=w620, "1D data"=w618, "append to file? (new file:F)"="append csv", "delimiter (\\t)"="," ("delimiter (\\t)")) -> ()  [unwired: 10 in, 2 out]
                }
              }
              n249 = Index Array(array=w572, index (row)="index (row)") -> ()  [unwired: 1 in, 1 out]
              "time" <- w573
            }
          }
        }
      }
      "name (unnamed) 2" <- w369
    }
    n250 = case shown="False" "RST" {
      tunnel: w262 -> [w358 _]
      tunnel: [w358 0] -> w285
      tunnel: [w357 w359] -> w283
      tunnel: w263 -> [w357 _]
      frame False {
      }
      frame True {
        n251 = Get Date/Time In Seconds() -> (seconds since 1Jan1904=w359:timestamp)
      }
    }
  }
  "error out 2" <- w69
  n252 = Close File(refnum=w61, error in=w88) -> (error out=→"error out":errorcluster)  [unwired: 1 out]
  n253 = call-poly <vilib>:"Write Delimited Spreadsheet.vi"("file path (dialog if empty)"=w72, "2D data"=w73, "append to file? (new file:F)"=FALSE, "transpose? (no:F)"=TRUE, "delimiter (\\t)"="," ("delimiter (\\t)")) -> ()  [unwired: 9 in, 2 out]
